vi "User Authentication List.vi"(7 "Username":string, 8 "Error In":errorcluster, 11 "Session In":refnum<class "Session.lvclass">) -> (0 "Error Out":errorcluster, 2 "List":string[](array[string]), 3 "Sesssion Out":refnum<class "Session.lvclass">)   [LabVIEW 2017, in "LabSSH2.lvlib" / "Session.lvclass"]
uses:
  Session.lvclass
  Session.lvclass/Session.ctl
  <vilib>/Utility/error.llb/Error Cluster From Error Code.vi
  <vilib>/ErrorRing/Error Ring.xnode
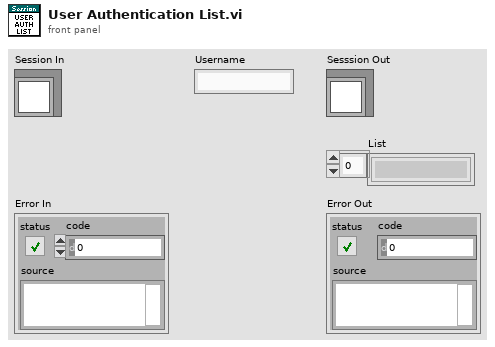
[diagram p1: front panel]
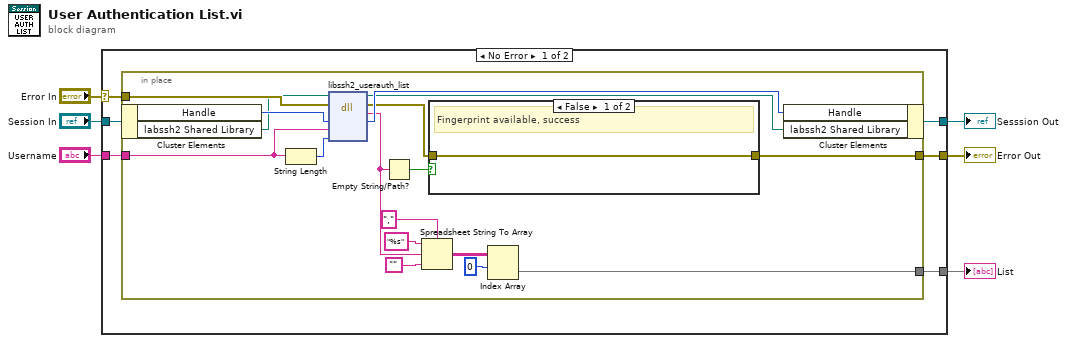
[diagram p0: block diagram]
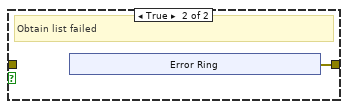
[diagram p2: hidden frame]
diagram:
  n1 = case shown="No Error" "Error In" {
    selector: "Error In" -> [w11 w37]
    tunnel: [w12 w37] -> w5
    tunnel: "Session In" -> [w10 w36]
    tunnel: [w9 w36] -> w3
    tunnel: "Username" -> [w8 _]
    tunnel: [w7 _] -> w1
    frame No Error {
      n2 = in-place {
        in-place-border: [w25] -> w12
        in-place-border: w11 -> [w24]
        in-place-border: w8 -> [w22]
        in-place-border: [w14] -> w7
        n3 = in-place-cluster #1(w10) -> ("Handle"=w29:u64, "labssh2 Shared Library"=w23:path)
        n4 = String Length(string=w22) -> (length=w21:i32)
        n5 = dll-call lib="D:/Users/cfield/Code/Field R&D Services/SSH/LabSSH2/LabVIEW/trunk/src/LabSSH2/Private/labssh2.*" fn="libssh2_userauth_list"(path in=w23, error in=w24, "session"=w29, "username"=w22, "username_len"=w21) -> (path out=w27:path, error out=w26:errorcluster, "List"=w18:string, "session"=w28:u64)  [unwired: 3 in]
        n6 = Empty String/Path?(string/path=w18) -> (empty?=w20:bool)
        n7 = Spreadsheet String To Array(delimiter (Tab)=",", format string="%s", spreadsheet string=w18, array type (2D Dbl)="") -> (array=w16:string[][])
        n8 = case shown="False" w20 {
          tunnel: w26 -> [w30 _]
          tunnel: [w30 w31] -> w25
          frame False {
            # "Fingerprint available, success"
          }
          frame True {
            # "Obtain list failed"
            n9 = xnode "Error Ring"() -> ("error out"=w31:errorcluster)
          }
        }
        n10 = Index Array(array=w16, index (row)=0) -> (element=w14:string[])  [unwired: 1 in]
        n11 = in-place-cluster #1("Handle"=w28, "labssh2 Shared Library"=w27) -> (w9:refnum<class "Session.lvclass">)
      }
    }
    frame Error {
    }
  }
  "Sesssion Out" <- w3
  "Error Out" <- w5
  "List" <- w1
